vi "FPGA Main.vi"() -> ()   [LabVIEW 2013]
doc: "This FPGA Main VI contains a control loop running in parallel with an RT watchdog loop.\n- The Control Loop performs control calculations on four input channels in parallel, and outputs the results to four output channels.\n- The RT Watchdog Loop checks for a periodic 'pet' from the RT Main VI to ensure communications between RT and FPGA are maintained."
uses:
  controls/FPGA State.ctl
  controls/Control Configuration.ctl
  controls/Raw Values.ctl
  <vilib>/LabVIEW Targets/FPGA/cRIO/cRIO-9505/controls.llb/_nicrio_cRIO-9505_DriveStatus.ctl
  controls/Custom Controller Inputs.ctl
  <vilib>/Platform/TimedLoop/XDataNode/timing_clust.ctl
  <vilib>/Platform/TimedLoop/XDataNode/nitl_modes.ctl
  <vilib>/Platform/TimedLoop/XDataNode/wakeup.ctl
  <vilib>/LabVIEW Targets/FPGA/cRIO/cRIO-9505/controls.llb/_nicrio_cRIO-9505_DriveDirection.ctl
  <vilib>/rvi/Emulation/niFpgaSctlEmulationGetInTimedLoop.vi
  <vilib>/rvi/Emulation/niFpgaEmulationReportErrorSimple.vi
  <vilib>/rvi/Emulation/niFpgaGetClockAttributes.vi
  <vilib>/rvi/Emulation/niFpgaCriticalErrorInLSC.vi
  <vilib>/rvi/Emulation/niFpgaProcessEmulError.vi
  <vilib>/rvi/eio/common/nirviEmuTemplateMethod_errors.vi
  <vilib>/rvi/eio/common/nirviEmuTemplatePropertyGet_noerrors.vi
  <vilib>/Platform/TimedLoop/XDataNode/XDataNode.xnode
  <vilib>/eio/EIONode/EIONode.xnode
  <vilib>/eio/EIOMethodNode/EIOMethodNode.xnode
  <vilib>/eio/EIOPropertyNode/EIOPropertyNode.xnode
  <vilib>/Platform/TimedLoop/XDataNode/XDNodeRunTimeDep.lvlib
  <vilib>/rvi/eio/common/nirviEmuTemplatePropertyGet_errors.vi
  <vilib>/rvi/eio/common/nirviEmuTemplatePropertySet_errors.vi
  <vilib>/rvi/eio/common/nirviEmuTemplatePropertySet_noerrors.vi
panel:
  in  "Custom Controller Inputs":T1={"Other Controller Gains"={"Position Control Kp"=0.0, "Virtual Spring Constant (N/m)"=3000.0, "Offset weight (N)"=0.5, "Fthresh (N)"=1.0, "Var2"=0.0}}
  in  "Mod1/AO4":fxp<+,16,3>
  in  "Trig AI":bool
  out "Vsup Present":bool
  out "Drive Fault":bool
  out "Drive Status":T2=enum."Disabled"
  out "Temp Fault":bool
  in  "Enable\nDrive":bool
  in  "Disable\nDrive":bool
  out "PWM Duty Cycle":i16
  out "F_Error (N)":fxp<+/-,40,11>
  in  "Force Sensor Gain (N/V)":fxp<+,20,6>=53.02703857421875
  in  "L12 Offset (mA)":fxp<+,18,4>=1.0
  in  "L12 Gain (mA/N)":fxp<+,16,2>=1.0
  out "Measured Force (N)":fxp<+,39,10>
  out "Controller\nOutput":fxp<+,18,3>
  in  "Channel 3 Setpoint":fxp<+/-,16,7>
  in  "Channel 2 Setpoint":fxp<+/-,20,7>
  in  "Channel 1 Setpoint  (Position)":fxp<+/-,20,7>=25.0
  in  "Channel 0 Setpoint (Force)":fxp<+/-,20,7>
  out "Watchdog Timed Out?":bool=TRUE
  in  "Enable Watchdog":bool
  in  "Pet Watchdog":bool
  in  "Watchdog Timeout Period (ticks)":u64=40000000 format="%.0p"
  out "Time Since Last Pet":u64
  in  "Manual Values":T3
  out "Output Values":T3
  out "Input Values":T3
  in  "Channel 3 Configuration":T4={"PID Gains"={"proportional gain (Kc)"=0.0, "integral gain (Kc*Ts/Ti)"=0.0, "derivative gain (Kc*Td/Ts)"=0.0}, "Output Range"={"output high"=10.0, "output low"=-10.0}}
  in  "Channel 2 Configuration":T4={"PID Gains"={"proportional gain (Kc)"=0.0, "integral gain (Kc*Ts/Ti)"=0.0, "derivative gain (Kc*Td/Ts)"=0.0}, "Output Range"={"output high"=10.0, "output low"=-10.0}}
  in  "Channel 1 Configuration":T4={"PID Gains"={"proportional gain (Kc)"=0.0, "integral gain (Kc*Ts/Ti)"=0.0, "derivative gain (Kc*Td/Ts)"=0.0}, "Output Range"={"output high"=10.0, "output low"=-10.0}}
  in  "Channel 0 Configuration":T4={"PID Gains"={"proportional gain (Kc)"=55.0, "integral gain (Kc*Ts/Ti)"=0.0, "derivative gain (Kc*Td/Ts)"=0.0}, "Output Range"={"output high"=50.0, "output low"=-50.0}}
  in  "New State":T5=enum."Control (PID)"
  out "Actual Loop Period (ticks)":u32
  out "Current FPGA State":T5=enum."Manual"
  in  "Change State":bool
  out "Input Error":bool
  out "Output Error":bool
  in  "Control Period (ticks)":u32
  # "General Settings"
  # "Manual Settings"
  # "Monitoring Values"
  # "Watchdog Settings"
  # "Control Settings"
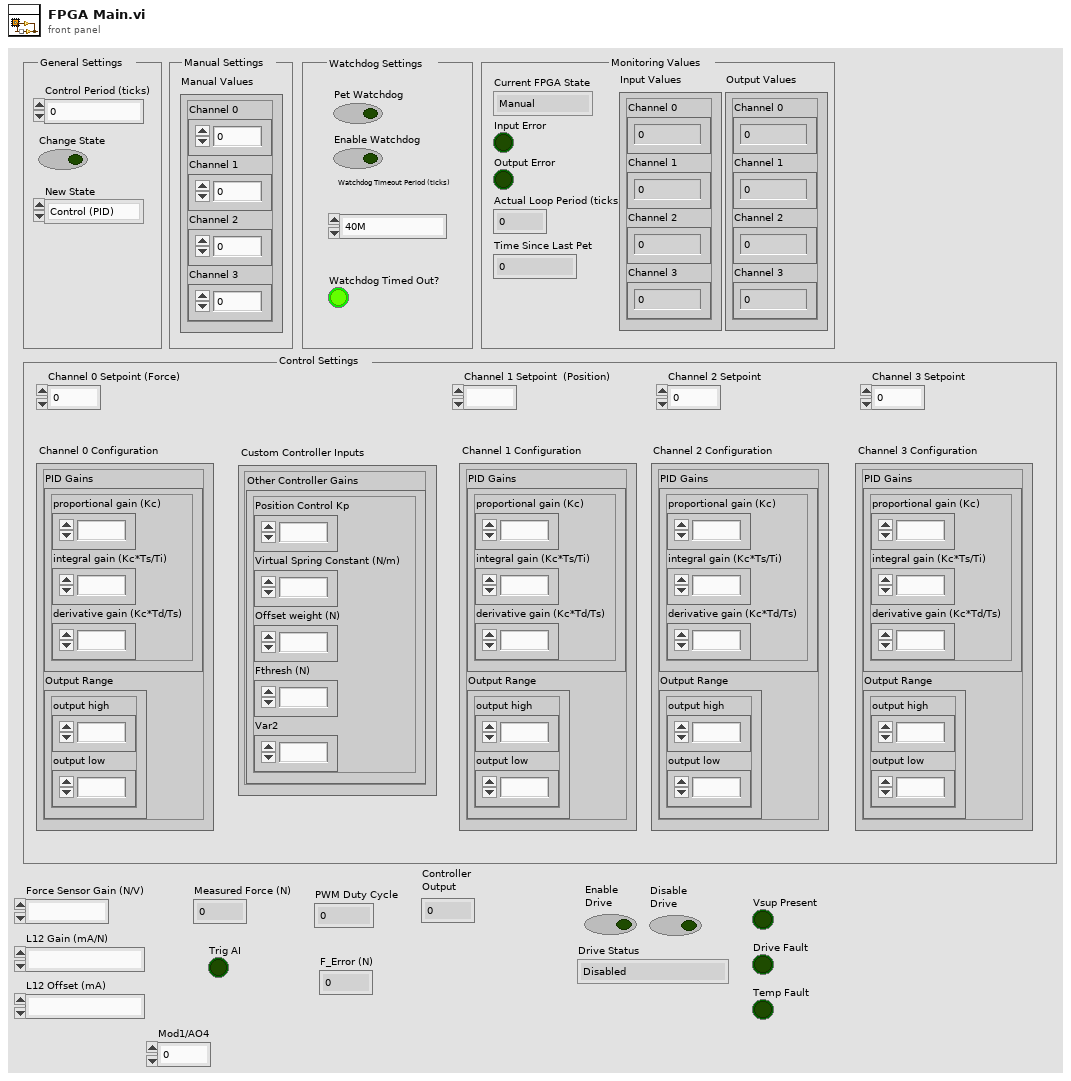
[diagram p1: front panel]
types:
  T1 = typedef "Custom Controller Inputs.ctl" = cluster{"Other Controller Gains":cluster{"Position Control Kp":fxp<+/-,16,8>, "Virtual Spring Constant (N/m)":fxp<+,16,12>, "Offset weight (N)":fxp<+/-,16,8>, "Fthresh (N)":fxp<+/-,16,5>, "Var2":fxp<+/-,16,5>}}
  T2 = typedef "_nicrio_cRIO-9505_DriveStatus.ctl" = enum8{"Enabled", "Disabled", "Disabled by Drive Fault", "Disabled by Temp. Fault", "Disabled by E-Stop", "Unknown"}
  T3 = typedef "Raw Values.ctl" = cluster{"Channel 0":fxp<+/-,20,7>, "Channel 1":fxp<+/-,20,7>, "Channel 2":fxp<+/-,20,7>, "Channel 3":fxp<+/-,20,14>}
  T4 = typedef "Control Configuration.ctl" = cluster{"PID Gains":cluster{"proportional gain (Kc)":fxp<+/-,16,8>, "integral gain (Kc*Ts/Ti)":fxp<+/-,16,8>, "derivative gain (Kc*Td/Ts)":fxp<+/-,16,8>}, "Output Range":cluster{"output high":fxp<+/-,16,7>, "output low":fxp<+/-,16,7>}}
  T5 = typedef "FPGA State.ctl" = enum16{"Safe State", "Manual", "Control (PID)"}
  T6 = typedef "XDNodeRunTimeDep.lvlib/timing_clust.ctl" = cluster{"Expected End [f-1]":u64, "Actual End [f-1]":u64, "Finished Late? [f-1]":bool, "Expected End [i-1]":u64, "Actual End [i-1]":u64, "Finished Late? [i-1]":bool, "Expected Start [i]":u64, "Actual Start [i]":u64, "Expected Start [f]":u64, "Actual Start [f]":u64, "Source Name":string, "Structure Name":string, "Period":i64, "Deadline":i64, "Offset":i64, "Start":i64, "Priority":i32, "Timeout":i32, "Mode":T7, "Wakeup Reason":T8, "Error":errorcluster, "Source Type":string, "Secondary Source Type":string, "Global End Time":u64, "Global Start Time":u64, "Frame Duration":u64, "Iteration Duration":u64, "Assigned CPU":i32, "I/O Scan Engine Mode":u32}
  T7 = typedef "XDNodeRunTimeDep.lvlib/nitl_modes.ctl" = enum32{"No Change", "Process missed periods, maintain original phase", "Discard missed periods, maintain original phase", "Process missed periods, ignore original phase", "Discard missed periods, ignore original phase"}
  T8 = typedef "XDNodeRunTimeDep.lvlib/wakeup.ctl" = enum32{"Normal", "Aborted", "Asynchronous wakeup", "Timing source error", "Timed loop error", "Timeout"}
  T9 = typedef "_nicrio_cRIO-9505_DriveDirection.ctl" = enum8{"Clockwise", "Counterclockwise"}
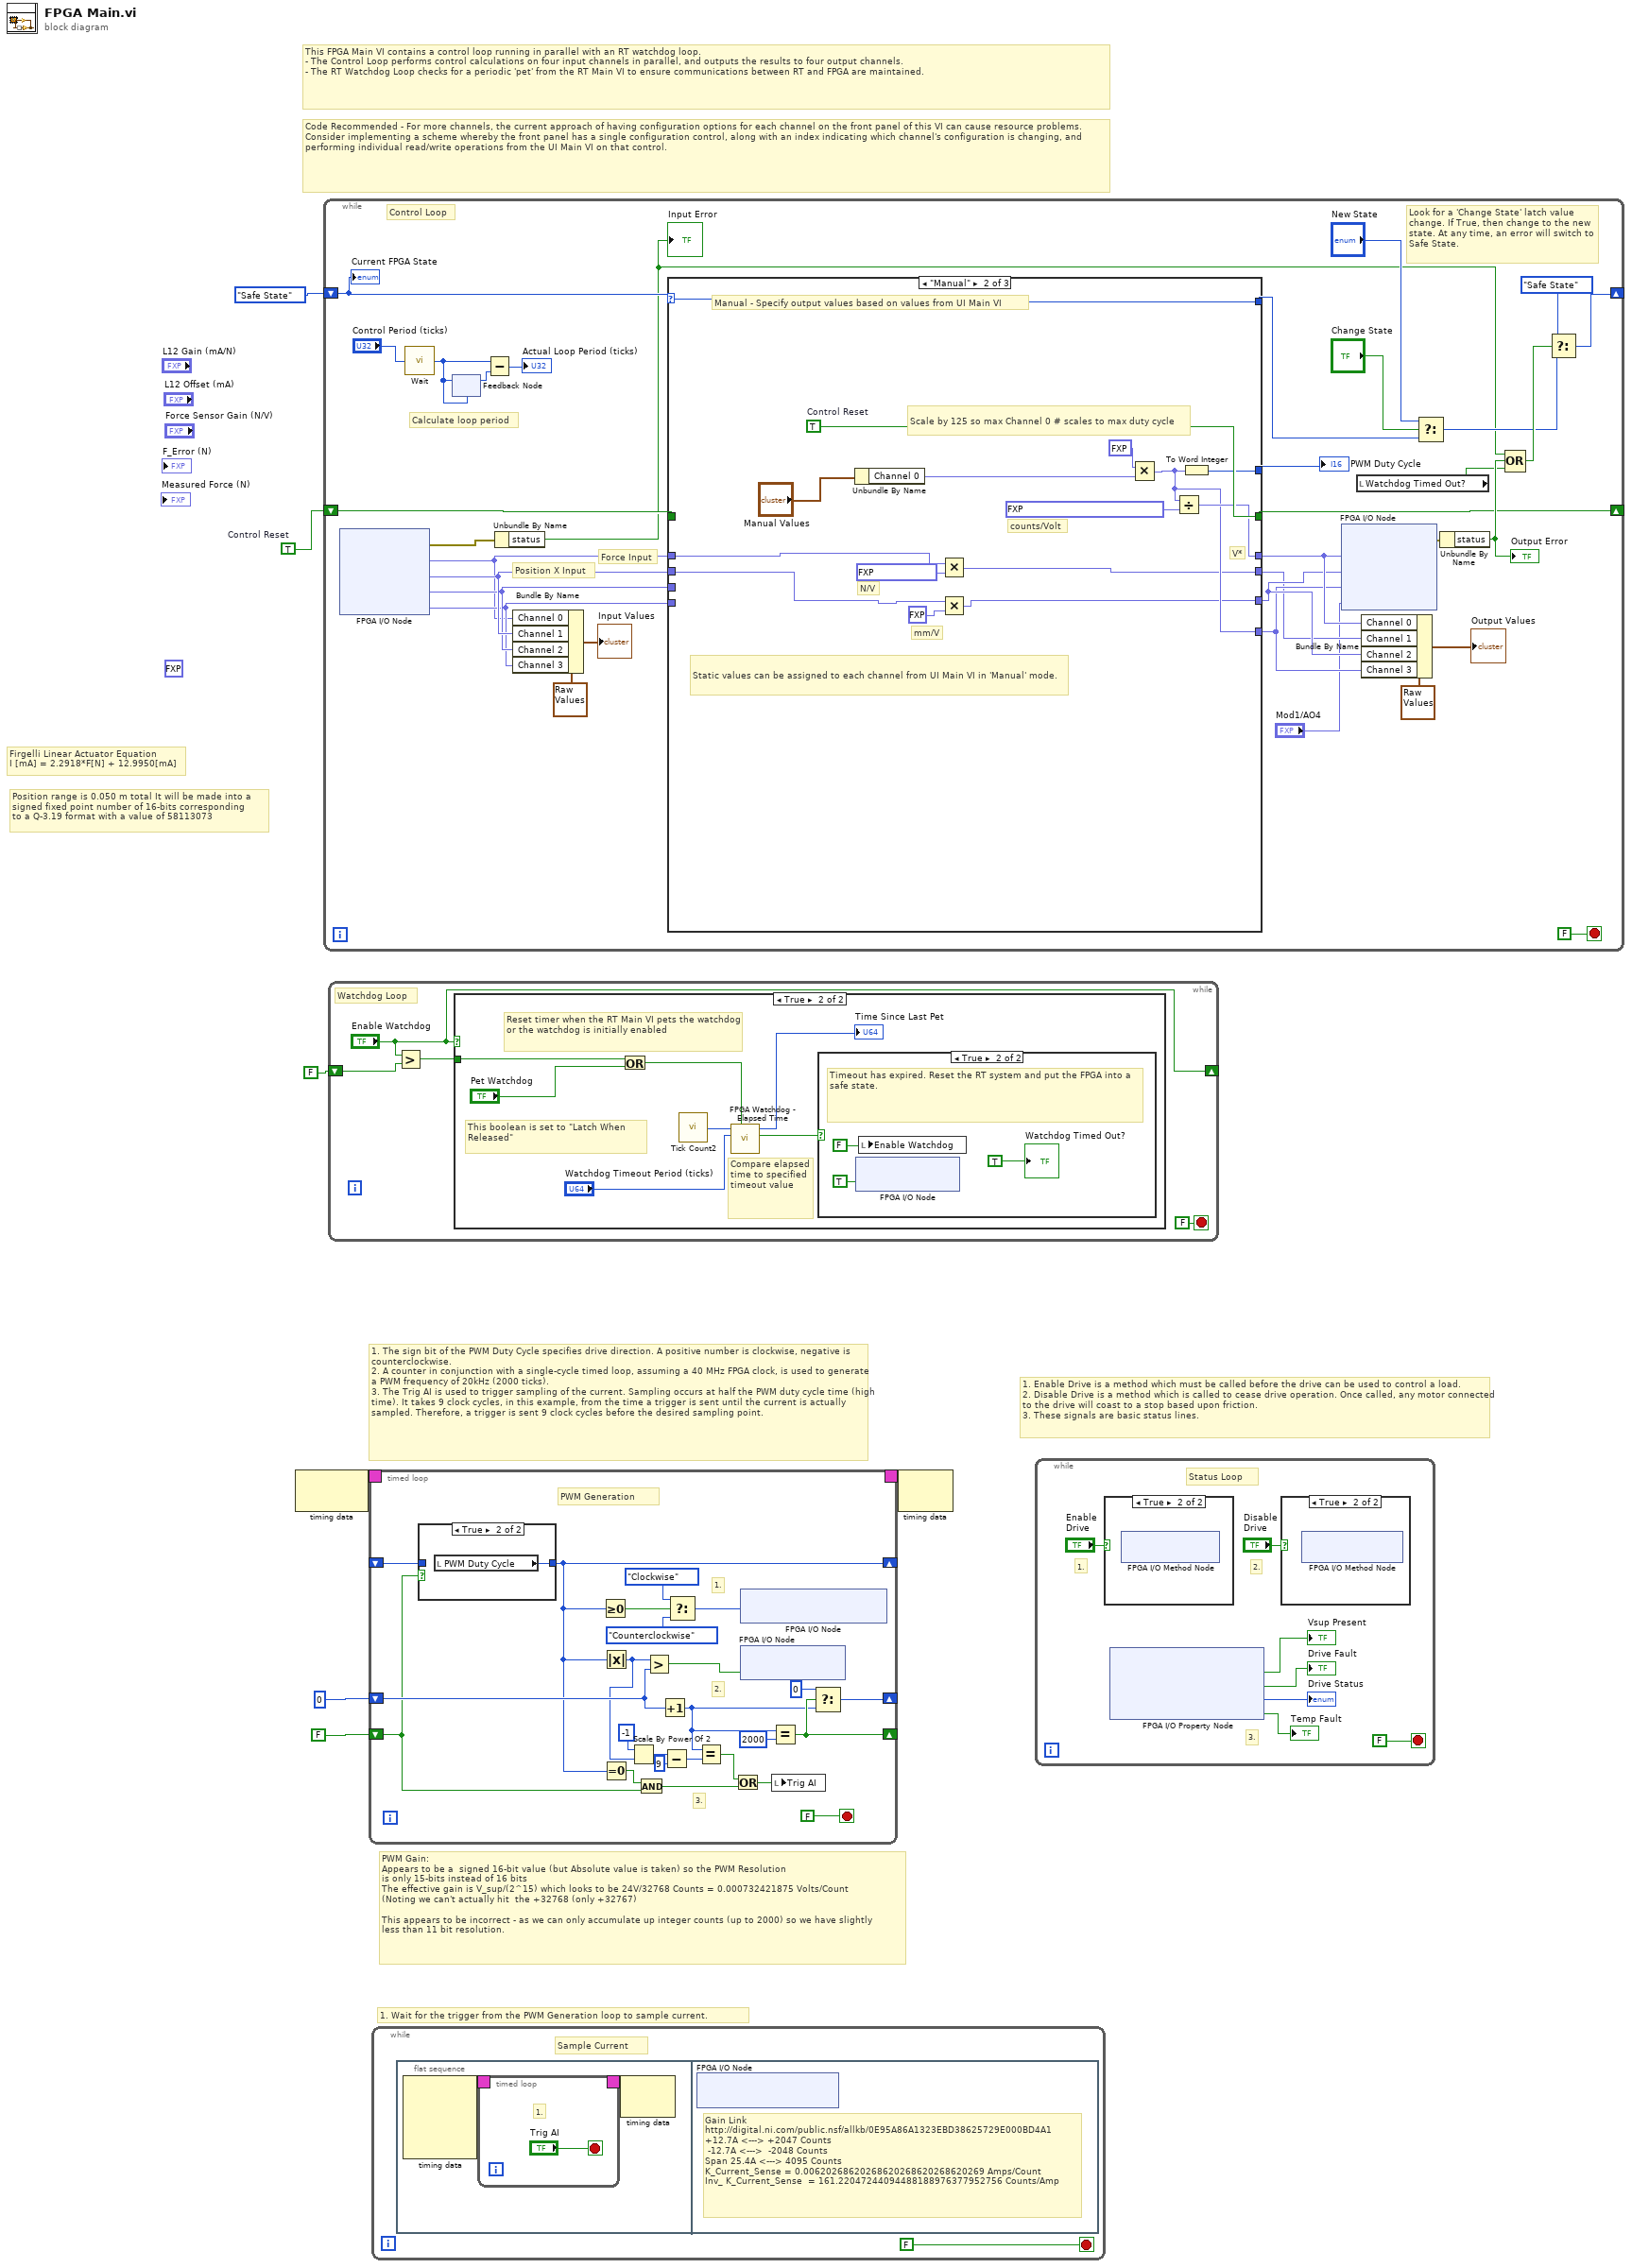
[diagram p0: block diagram]
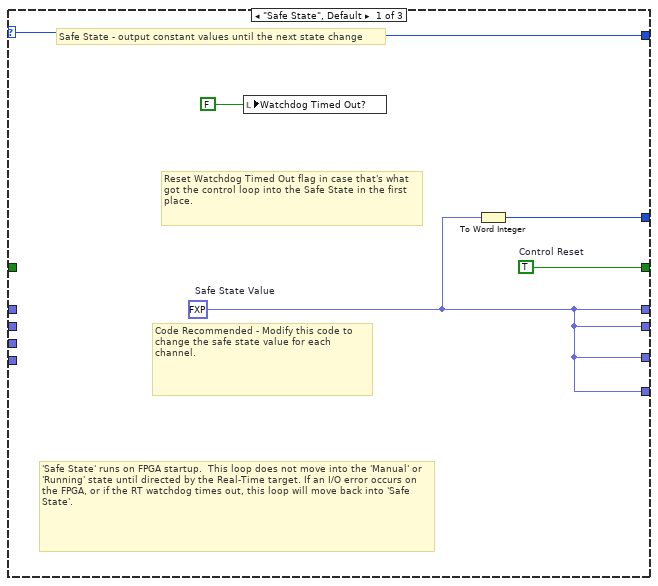
[diagram p7: hidden frame]
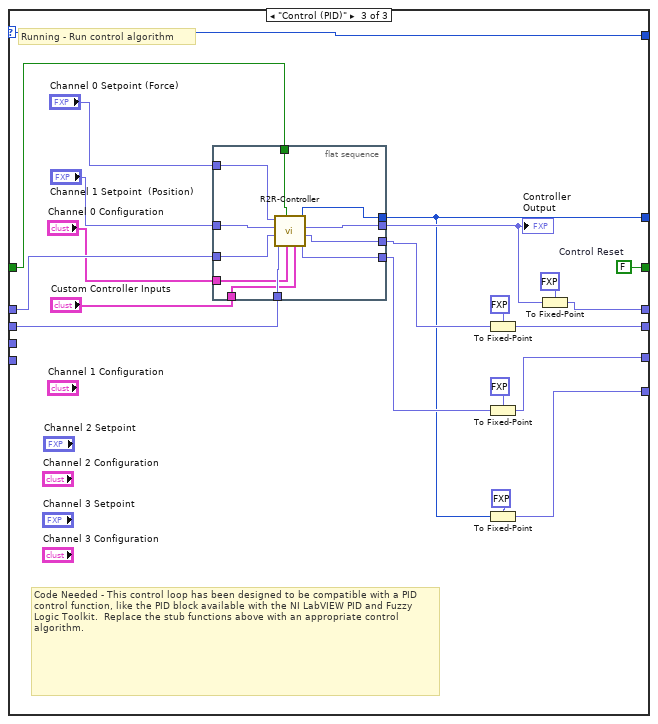
[diagram p8: hidden frame]
diagram:
  (unwired) fxp<+,18,3> 0.0 ("F (Raw Analog V)")
  w6 = TRUE  # Control Reset
  # "PWM Gain:\nAppears to be a  signed 16-bit value (but Absolute value is taken) so the PWM Resolution\nis only 15-bits instead of 16 bits\nThe effective gain is V_sup/(2^15) which looks to be 24V/32768 Counts = 0.000732421875 Volts/Count\n(Noting we can't actually hit  the +32768 (only +32767)\n\nThis appears to be incorrect - as we can only accumulate up integer counts (up to 2000) so we have slightly\nless than 11 bit resolution."
  # "1. Enable Drive is a method which must be called before the drive can be used to control a load.\n2. Disable Drive is a method which is called to cease drive operation. Once called, any motor connected to the drive will coast to a stop based upon friction.\n3. These signals are basic status lines."
  # "1. Wait for the trigger from the PWM Generation loop to sample current."
  # "1. The sign bit of the PWM Duty Cycle specifies drive direction. A positive number is clockwise, negative is counterclockwise.\n2. A counter in conjunction with a single-cycle timed loop, assuming a 40 MHz FPGA clock, is used to generate a PWM frequency of 20kHz (2000 ticks).\n3. The Trig AI is used to trigger sampling of the current. Sampling occurs at half the PWM duty cycle time (high time). It takes 9 clock cycles, in this example, from the time a trigger is sent until the current is actually sampled. Therefore, a trigger is sent 9 clock cycles before the desired sampling point."
  # "Position range is 0.050 m total It will be made into a \nsigned fixed point number of 16-bits corresponding \nto a Q-3.19 format with a value of 58113073"
  # "Firgelli Linear Actuator Equation\nI [mA] = 2.2918*F[N] + 12.9950[mA]"
  # "Code Recommended - For more channels, the current approach of having configuration options for each channel on the front panel of this VI can cause resource problems.  Consider implementing a scheme whereby the front panel has a single configuration control, along with an index indicating which channel's configuration is changing, and performing individual read/write operations from the UI Main VI on that control."
  # "This FPGA Main VI contains a control loop running in parallel with an RT watchdog loop.\n- The Control Loop performs control calculations on four input channels in parallel, and outputs the results to four output channels.\n- The RT Watchdog Loop checks for a periodic 'pet' from the RT Main VI to ensure communications between RT and FPGA are maintained."
  n1 = node-c288() -> (w4:T6)  [unwired: 1 out]
  n2 = while {
    shift-right: [w36] -> _
    shift-left: FPGA_State."Safe State" ("FPGA State") -> [w27]
    shift-right: [w33] -> _
    shift-left: w6 -> [w32]
    stop <- FALSE stop-if-true
    # "Position X Input"
    # "Force Input"
    # "Calculate loop period"
    # "Look for a 'Change State' latch value change. If True, then change to the new state. At any time, an error will switch to Safe State."
    # "Control Loop"
    n3 = xnode "FPGA I/O Node"() -> ("error out"=w40:errorcluster, "Mod1/AI0"=w10:fxp<+,18,3>, "Mod1/AI1"=w25:fxp<+,18,3>, "Mod1/AI2"=w24:fxp<+,18,3>, "Mod1/AI3"=w23:fxp<+,18,3>)  [unwired: 5 in, 4 out]
    n4 = call "Wait"("Count(Ticks)"="Control Period (ticks)") -> ("Tick Count(Ticks)"=w16:u32)
    n5 = feedback-in #1(w16) -> ()
    n6 = feedback #1(w16) -> (w15:u32)
    n7 = Subtract(x=w16, y=w15) -> (x-y=→"Actual Loop Period (ticks)":u32)
    n8 = Unbundle By Name(w40) -> ("status"=w26:bool)
    "Input Error" <- w26
    n9 = Bundle By Name(cluster=T3 {"Channel 0"=0.0, "Channel 1"=0.0, "Channel 2"=0.0, "Channel 3"=0.0} ("Raw Values"), "Channel 0"=w10, "Channel 1"=w25, "Channel 2"=w24, "Channel 3"=w23) -> (→"Input Values":T3)
    n10 = case shown="\"Manual\"" w27 {
      selector: w27 -> [w45 w60 w79]
      tunnel: w10 -> [_ w51 w69]
      tunnel: [w42 w54 w81] -> w22
      tunnel: [w45 w60 w79] -> w31
      tunnel: [w46 w61 w80] -> w33
      tunnel: w32 -> [_ _ w72]
      tunnel: w25 -> [_ w48 w66]
      tunnel: w24 -> [_ _ _]
      tunnel: w23 -> [_ _ _]
      tunnel: [w42 w50 w75] -> w11
      tunnel: [w42 w47 w74] -> w21
      tunnel: [w42 w53 w73] -> w20
      tunnel: [w43 w58 w63] -> w9
      frame "Safe State", Default {
        w42 = fxp<+/-,20,7> 0.0  # Safe State Value
        w46 = TRUE  # Control Reset
        # "'Safe State' runs on FPGA startup.  This loop does not move into the 'Manual' or 'Running' state until directed by the Real-Time target. If an I/O error occurs on the FPGA, or if the RT watchdog times out, this loop will move back into 'Safe State'."
        # "Reset Watchdog Timed Out flag in case that's what got the control loop into the Safe State in the first place."
        # "Safe State - output constant values until the next state change"
        # "Code Recommended - Modify this code to change the safe state value for each channel."
        n11 = local write "Watchdog Timed Out?"(FALSE ("Watchdog Timed Out?")) -> ()
        n12 = To Word Integer(number=w42) -> (16bit integer=w43:i16)
      }
      frame "Manual" {
        w61 = TRUE  # Control Reset
        # "N/V"
        # "mm/V"
        # "V*"
        # "counts/Volt"
        # "Scale by 125 so max Channel 0 # scales to max duty cycle"
        # "Manual - Specify output values based on values from UI Main VI"
        # "Static values can be assigned to each channel from UI Main VI in 'Manual' mode."
        n13 = Unbundle By Name("Manual Values") -> ("Channel 0"=w56:fxp<+/-,20,7>)
        n14 = Multiply(x=w51, y=fxp<+,20,6> 53.02685546875) -> (x*y=w50:fxp<+,38,9>)
        n15 = Multiply(x=w48, y=fxp<+,12,4> 10.0) -> (x*y=w47:fxp<+,30,7>)
        n16 = Multiply(x=fxp<+/-,20,8> 125.0, y=w56) -> (x*y=w53:fxp<+/-,40,15>)
        n17 = Divide(x=w53, y=fxp<+/-,40,15> 83.33199998736382) -> (x/y=w54:fxp<+/-,64,40>)
        n18 = To Word Integer(number=w53) -> (16bit integer=w58:i16)
      }
      frame "Control (PID)" {
        w80 = FALSE  # Control Reset
        # "Running - Run control algorithm"
        # "Code Needed - This control loop has been designed to be compatible with a PID control function, like the PID block available with the NI LabVIEW PID and Fuzzy Logic Toolkit.  Replace the stub functions above with an appropriate control algorithm."
        n19 = flat-sequence {
          tunnel: "Channel 0 Setpoint (Force)" -> [w92]
          tunnel: w72 -> [w93]
          tunnel: w69 -> [w90]
          tunnel: [w85] -> w71
          tunnel: "Channel 0 Configuration" -> [w88]
          tunnel: "Custom Controller Inputs" -> [w87]
          tunnel: "Channel 1 Setpoint  (Position)" -> [w91]
          tunnel: w66 -> [w89]
          tunnel: [w86] -> w63
          tunnel: [w84] -> w65
          tunnel: [w83] -> w64
          frame #0 {
            n20 = call "R2R-Controller.vi"("Custom Controller Inputs"=w87, "Gain Configuration"=w88, "Reset Integrator"=w93, "X (Raw Analog V)"=w89, "F (Raw Analog V)"=w90, "X* (mm)"=w91, "F* (N)"=w92) -> ("Xmeas (mm)"=w83:fxp<+/-,35,12>, "Fmeas (N)"=w84:fxp<+,39,10>, "V*(V)"=w85:fxp<+/-,53,13>, "PWM Duty Cycle"=w86:i16)  [unwired: 1 out]
          }
        }
        n21 = To Fixed-Point(fixed-point type=fxp<+/-,20,7> 0.0 ("Off Value"), number=w65) -> (fixed-point=w75:fxp<+/-,20,7>)
        n22 = To Fixed-Point(fixed-point type=fxp<+/-,20,7> 0.0 ("Off Value"), number=w64) -> (fixed-point=w74:fxp<+/-,20,7>)
        n23 = To Fixed-Point(fixed-point type=fxp<+/-,20,7> 0.0 ("Off Value"), number=w63) -> (fixed-point=w73:fxp<+/-,20,7>)
        n24 = To Fixed-Point(fixed-point type=fxp<+/-,20,7> 0.0 ("Off Value"), number=w71) -> (fixed-point=w81:fxp<+/-,20,7>)
        "Controller\nOutput" <- w71
      }
    }
    "PWM Duty Cycle" <- w9
    n25 = xnode "FPGA I/O Node"("Mod1/AO0"=w22, "Mod1/AO2"=w21, "Mod1/AO3"=w20, "Mod1/AO4"="Mod1/AO4") -> ("error out"=w39:errorcluster)  [unwired: 5 in, 4 out]
    n26 = local read "Watchdog Timed Out?"() -> (w17:bool)
    n27 = Bundle By Name(cluster=T3 {"Channel 0"=0.0, "Channel 1"=0.0, "Channel 2"=0.0, "Channel 3"=0.0} ("Raw Values"), "Channel 0"=w22, "Channel 1"=w11, "Channel 2"=w21, "Channel 3"=w20) -> (→"Output Values":T3)
    n28 = Select(t="New State", s="Change State", f=w31) -> (s? t:f=w28:T5)
    n29 = Unbundle By Name(w39) -> ("status"=w38:bool)
    "Output Error" <- w38
    n30 = Compound Arithmetic op=OR(w26, w38, w17) -> (w35:bool)
    n31 = Select(t=FPGA_State."Safe State" ("FPGA State"), s=w35, f=w28) -> (s? t:f=w36:T5)
    "Current FPGA State" <- w27
  }
  n32 = while "RT Watchdog Loop" {
    shift-right: ["Enable Watchdog"] -> _
    shift-left: FALSE ("Enable RT Watchdog") -> [w97]
    stop <- FALSE stop-if-true
    # "Watchdog Loop"
    n33 = Greater?(x="Enable Watchdog", y=w97) -> (0:w94:bool)
    n34 = case shown="True" "Enable Watchdog" {
      tunnel: w94 -> [_ w100]
      frame False {
        # "This loop has to be explicitly enabled from the RT Main VI.  This reduces the possiblity of an endless reboot cycle."
      }
      frame True {
        # "This boolean is set to \"Latch When Released\""
        # "Compare elapsed time to specified timeout value"
        # "Reset timer when the RT Main VI pets the watchdog or the watchdog is initially enabled"
        n35 = Or(x=w100, y="Pet Watchdog") -> (x .or. y?=w99:bool)
        n36 = call "Tick Count2"() -> ("Tick Count(Ticks)"=w103:u32)
        n37 = call "FPGA Watchdog - Elapsed Time.vi"("Reset"=w99, "Timeout Period"="Watchdog Timeout Period (ticks)", "Current Time"=w103) -> ("Timeout"=w98:bool, "Elapsed Time"=→"Time Since Last Pet":u64)  [unwired: 7 in]
        n38 = case shown="True" w98 {
          frame False {
            # "Timeout has not expired."
          }
          frame True {
            # "Timeout has expired. Reset the RT system and put the FPGA into a safe state."
            n39 = xnode "FPGA I/O Node"("System Reset"=TRUE ("RT Reset on Watchdog Failure?")) -> ()  [unwired: 1 in, 1 out]
            n40 = local write "Enable Watchdog"(FALSE ("Enable RT Watchdog")) -> ()
            "Watchdog Timed Out?" <- TRUE ("Watchdog Timed Out?")
          }
        }
      }
    }
  }
  n41 = timed-loop {
    timing: w4 -> [_]
    timing-out: [_] -> w3
    shift-right: [w128] -> _
    shift-left: i16 0 -> [w131]
    shift-right: [w127] -> _
    shift-left: FALSE -> [w124]
    shift-right: [w108] -> _
    shift-left: _ -> [w126]
    stop <- FALSE stop-if-true
    # "3."
    # "2."
    # "1."
    # "PWM Generation"
    n42 = case shown="True" w124 {
      tunnel: [w132 w133] -> w108
      tunnel: w126 -> [w132 _]
      frame False {
      }
      frame True {
        n43 = local read "PWM Duty Cycle"() -> (w133:i16)
      }
    }
    n44 = Greater Or Equal To 0?(x=w108) -> (x >= 0?=w120:bool)
    n45 = Absolute Value(x=w108) -> (abs(x)=w110:i16)
    n46 = Equal To 0?(x=w108) -> (x = 0?=w125:bool)
    n47 = Scale By Power Of 2(n=i8 -1, x=w110) -> (x*2^n=w113:i16)
    n48 = And(x=w125, y=w124) -> (x .and. y?=w121:bool)
    n49 = Greater?(x=w110, y=w131) -> (0:w117:bool)
    n50 = Increment(x=w131) -> (x+1=w123:i16)
    n51 = Subtract(x=w113, y=i8 9) -> (x-y=w112:i16)
    n52 = Select(t=_nicrio_cRIO-9505_DriveDirection."Clockwise" ("Drive Direction"), s=w120, f=_nicrio_cRIO-9505_DriveDirection."Counterclockwise" ("Drive Direction")) -> (s? t:f=w116:T9)
    n53 = Equal?(x=w123, y=w112) -> (x = y?=w122:bool)
    n54 = Or(x=w122, y=w121) -> (x .or. y?=w115:bool)
    n55 = xnode "FPGA I/O Node"("Mod2/Drive Direction"=w116) -> ()  [unwired: 1 in, 1 out]
    n56 = xnode "FPGA I/O Node"("Mod2/Motor"=w117) -> ()  [unwired: 1 in, 1 out]
    n57 = Equal?(x=w123, y=i16 2000) -> (x = y?=w127:bool)
    n58 = local write "Trig AI"(w115) -> ()
    n59 = Select(t=i16 0, s=w127, f=w123) -> (s? t:f=w128:i16)
  }
  n60 = while {
    stop <- FALSE stop-if-true
    # "Sample Current"
    n61 = flat-sequence {
      frame #0 {
        n62 = node-c288() -> (w138:T6)  [unwired: 4 out]
        n63 = timed-loop {
          timing: w138 -> [_]
          timing-out: [_] -> w137
          stop <- "Trig AI" stop-if-true
          # "1."
        }
        n64 = node-c288(w137) -> ()  [unwired: 1 out]
      }
      frame #1 {
        # "Gain Link\nhttp://digital.ni.com/public.nsf/allkb/0E95A86A1323EBD38625729E000BD4A1\n+12.7A <---> +2047 Counts\n -12.7A <--->  -2048 Counts\nSpan 25.4A <---> 4095 Counts\nK_Current_Sense = 0.00620268620268620268620268620269 Amps/Count\nInv_ K_Current_Sense  = 161.22047244094488188976377952756 Counts/Amp"
        n65 = xnode "FPGA I/O Node"() -> ()  [unwired: 1 in, 2 out]
      }
    }
  }
  n66 = node-c288(w3) -> ()  [unwired: 1 out]
  n67 = while {
    stop <- FALSE stop-if-true
    # "3."
    # "2."
    # "1."
    # "Status Loop"
    n68 = case shown="True" "Enable\nDrive" {
      frame False {
      }
      frame True {
        n69 = xnode "FPGA I/O Method Node"() -> ()  [unwired: 1 in, 1 out]
      }
    }
    n70 = xnode "FPGA I/O Property Node"() -> ("Vsup Present"=→"Vsup Present":bool, "Drive Fault"=→"Drive Fault":bool, "Drive Status"=→"Drive Status":T2, "Over Temperature Fault"=→"Temp Fault":bool)  [unwired: 1 in, 1 out]
    n71 = case shown="True" "Disable\nDrive" {
      frame False {
      }
      frame True {
        n72 = xnode "FPGA I/O Method Node"() -> ()  [unwired: 1 in, 1 out]
      }
    }
  }
